vi "Upload to S3.vi"(8 "error in (no error)":errorcluster, 10 "file to upload":path, 11 "Control Experiment in":refnum<class "Control Experiment.lvclass">) -> (0 "error out":errorcluster)   [LabVIEW 2016, in "Control Experiment.lvclass"]
uses:
  Control Experiment.lvclass
  Control Experiment.lvclass/Control Experiment.ctl
  <userlib>/LevyLab/postgreSQL-timescaleDB/Data.S3/Data.S3.lvclass
panel:
  out "Object Path":string
  out "Control Experiment out":refnum<class "Control Experiment.lvclass">
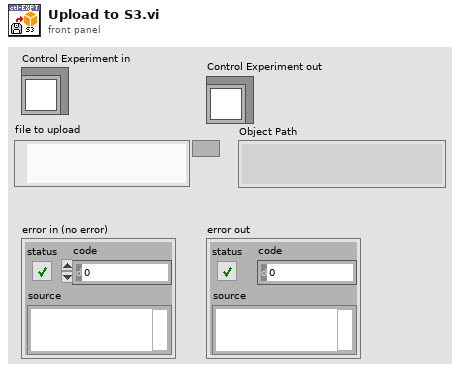
[diagram p1: front panel]
types:
  T1 = typedef "Control Experiment.lvclass/Instrument--enum.ctl" = enum16{"----- AFM/EBL -----", "AGILENT", "CYPHER", "Gemini2", "JEOL", "MFP3D", "----- Cryostat -----", "CF900", "DR200", "MNK", "PPMS 1", "PPMS 2", "PPMS 3", "----- Optics -----", "THz 1 (Element 2/Montana)", "THz 2 (Tsunami/Janis)"}
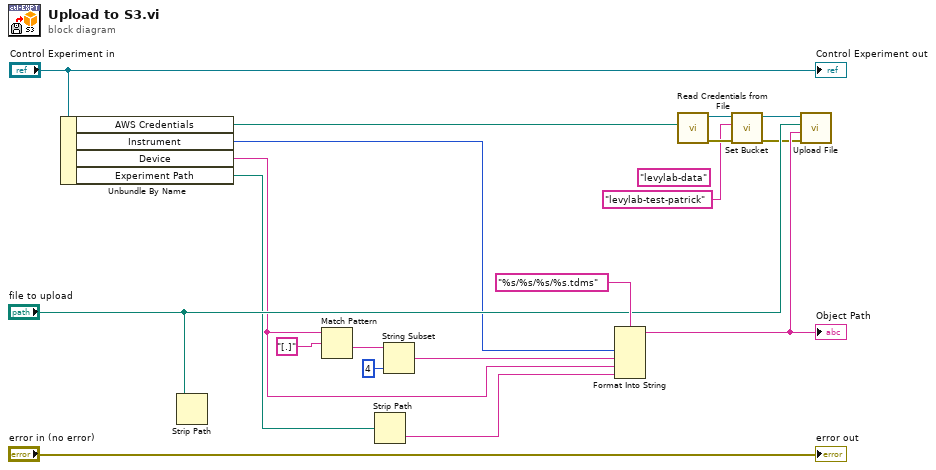
[diagram p0: block diagram]
diagram:
  (unwired) "levylab-data" ("Bucket name")
  n1 = Unbundle By Name("Control Experiment in") -> ("AWS Credentials"=w2:path, "Instrument"=w10:T1, "Device"=w11:string, "Experiment Path"=w4:path)
  n2 = Strip Path(path="file to upload") -> ()  [unwired: 2 out]
  n3 = Match Pattern(string=w11, regular expression="[.]" ("delimiter (Tab)")) -> (after substring=w12:string)  [unwired: 1 in, 3 out]
  n4 = Strip Path(path=w4) -> (name=w3:string)  [unwired: 1 out]
  n5 = String Subset(string=w12, length (rest)=4 ("length (rest)")) -> (substring=w16:string)  [unwired: 1 in]
  n6 = Format Into String(format string="%s/%s/%s/%s.tdms", w10, w16, w11, w3) -> (resulting string=w14:string)  [unwired: 2 in, 1 out]
  "Object Path" <- w14
  n7 = call <userlib>:"Read Credentials from File.vi"("path to aws credentials"=w2) -> ("error out"=w9:errorcluster, "Data.S3 out"=w8:refnum<class "Data.S3.lvclass">)  [unwired: 9 in]
  n8 = call <userlib>:"Set Bucket.vi"("error in (no error)"=w9, "Bucket name"="levylab-test-patrick", "Data.S3"=w8) -> ("error out"=w6:errorcluster, "Data.S3"=w7:refnum<class "Data.S3.lvclass">)  [unwired: 7 in]
  n9 = call <userlib>:"Upload File.vi"("error in (no error)"=w6, "Object Path (including file name)"=w14, "file to upload"="file to upload", "Data.S3"=w7) -> ()  [unwired: 6 in, 2 out]
  "error out" <- "error in (no error)"
  "Control Experiment out" <- "Control Experiment in"
